vi "Mcp2210 Enter Password.vi"(8 "error in (no error)":errorcluster, 10 "passwd":string, 11 "handle":i32) -> (0 "error out":errorcluster, 2 "passwd out":string, 3 "handle out":i32)   [LabVIEW 2015, in "mcp2210.lvlib"]
doc: "Sends the NVRAM unlock password to the device.\nThe function returns 0 (M_E_SUCCESS) either if the password is accepted or if the device is not\npassword protected. In both cases, the NVRAM changes are permitted.\nThe function returns negative error code in case of device communication failure or if the password\nis not accepted by the device.\nRejected password error codes:\n- M_E_ERR_NVRAM_LOCKED - NVRAM is permanently locked, no password is accepted\n- M_E_ERR_WRONG_PASSWD - password mismatch, but number of attempts is less than 5\n- M_E_ERR_ACCESS_DENIED - password mismatch, but the number of attempts exceeded 5,\nso the NVRAM writes are blocked until the next device reset\nParameters:\nInputs:\n- IntPtr handle - The USB device handle. Cannot be NULL.\n- String ^passwd - string of 8 characters. Cannot be NULL.\n!!! Important !!!\nThe password must have exactly 8 characters. If there is a different\nnumber of characters, -2 (M_E_ERR_INVALID_PARAMETER) error code is returned.\nThe String UNICODE characters are converted to ANSI string before being sent\nto the device for verification.\nOutputs:\n- none\nReturns:\n- 0 for success: M_E_SUCCESS\n- negative error code: M_E_ERR_NULL, M_E_ERR_INVALID_HANDLE_VALUE, M_E_ERR_INVALID_PARAMETER\nM_E_ERR_HID_TIMEOUT, M_E_ERR_HID_RW_FILEIO, M_E_ERR_UNKOWN_ERROR\nM_E_ERR_NVRAM_LOCKED, M_E_ERR_WRONG_PASSWD, M_E_ERR_ACCESS_DENIED\nM_E_ERR_CMD_ECHO, M_E_ERR_CMD_FAILED\n\nMCP2210_DLL_UM_API int __stdcall Mcp2210_EnterPassword(void *handle, char *passwd);"
uses:
  <userlib>/mcp2210/mcp2210.lvlib
  <userlib>/mcp2210/mcp2210_dll_um_x86.dll
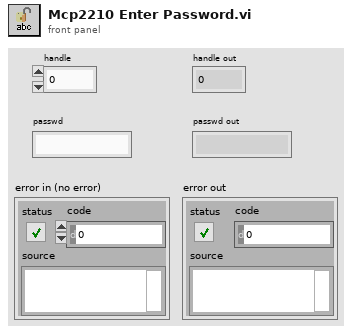
[diagram p1: front panel]
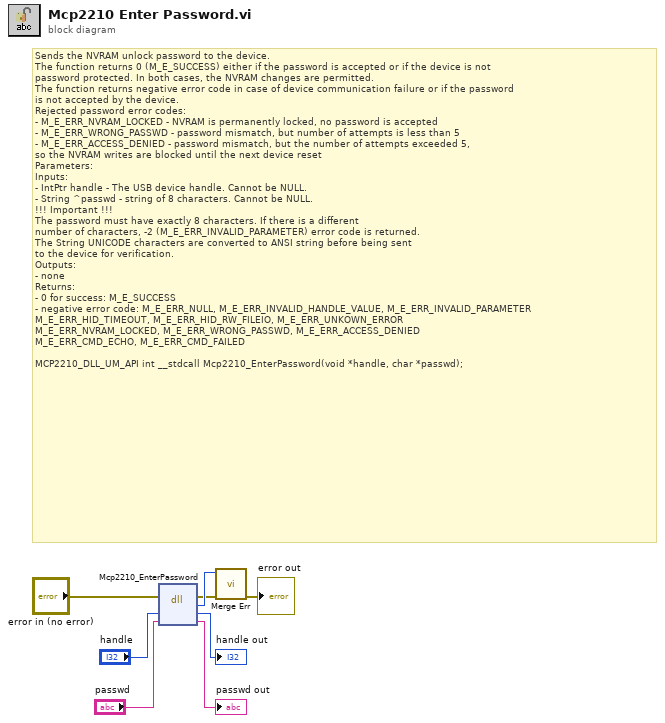
[diagram p0: block diagram]
diagram:
  # "Sends the NVRAM unlock password to the device.\nThe function returns 0 (M_E_SUCCESS) either if the password is accepted or if the device is not\npassword protected. In both cases, the NVRAM changes are permitted.\nThe function returns negative error code in case of device communication failure or if the password\nis not accepted by the device.\nRejected password error codes:\n- M_E_ERR_NVRAM_LOCKED - NVRAM is permanently locked, no password is accepted\n- M_E_ERR_WRONG_PASSWD - password mismatch, but number of attempts is less than 5\n- M_E_ERR_ACCESS_DENIED - password mismatch, but the number of attempts exceeded 5,\nso the NVRAM writes are blocked until the next device reset\nParameters:\nInputs:\n- IntPtr handle - The USB device handle. Cannot be NULL.\n- String ^passwd - string of 8 characters. Cannot be NULL.\n!!! Important !!!\nThe password must have exactly 8 characters. If there is a different\nnumber of characters, -2 (M_E_ERR_INVALID_PARAMETER) error code is returned.\nThe String UNICODE characters are converted to ANSI string before being sent\nto the device for verification.\nOutputs:\n- none\nReturns:\n- 0 for success: M_E_SUCCESS\n- negative error code: M_E_ERR_NULL, M_E_ERR_INVALID_HANDLE_VALUE, M_E_ERR_INVALID_PARAMETER\nM_E_ERR_HID_TIMEOUT, M_E_ERR_HID_RW_FILEIO, M_E_ERR_UNKOWN_ERROR\nM_E_ERR_NVRAM_LOCKED, M_E_ERR_WRONG_PASSWD, M_E_ERR_ACCESS_DENIED\nM_E_ERR_CMD_ECHO, M_E_ERR_CMD_FAILED\n\nMCP2210_DLL_UM_API int __stdcall Mcp2210_EnterPassword(void *handle, char *passwd);"
  n1 = dll-call lib="D:/LabVIEW 2015/user.lib/mcp2210/mcp2210_dll_um_x86.*" fn="Mcp2210_EnterPassword"(error in="error in (no error)", "handle"="handle", "passwd"="passwd") -> (error out=w3:errorcluster, "return type"=w4:i32, "handle"=→"handle out":i32, "passwd"=→"passwd out":string)  [unwired: 2 in, 1 out]
  n2 = call <userlib>:"Merge Err.vi"("error in (no error)"=w3, "return type"=w4) -> ("error out"=→"error out":errorcluster)  [unwired: 9 in]
